vi "dds_reset.vi"(4 "constants in":T3, 7 "counter in":u8, 8 "FPGA parameters in":T2 {"y-point bandwidth" format="%.28g"; "x-point bandwidth" format="%.28g"; "AOD center frequ. (Hz)_y" format="%.14g"; "AOD half bandwidth_y" format="%.14g"; "AOD Bandwidth_y (Hz)" format="%_6f"; "AOD center frequ. (Hz)_x" format="%.14g"; "cos Phi" format="%.35g"; "sin Phi" format="%.35g"; "AOD_Scale_Factor (1/Zoom)" format="%.35g"; "AOD half bandwidth_x" format="%.14g"; "AOD Bandwidth_x (Hz)" format="%_6f"}, 9 "reset dds in":bool=TRUE, 10 "FPGA parameters after reset":T2 {"y-point bandwidth" format="%.28g"; "x-point bandwidth" format="%.28g"; "AOD center frequ. (Hz)_y" format="%.14g"; "AOD half bandwidth_y" format="%.14g"; "AOD Bandwidth_y (Hz)" format="%_6f"; "AOD center frequ. (Hz)_x" format="%.14g"; "cos Phi" format="%.35g"; "sin Phi" format="%.35g"; "AOD_Scale_Factor (1/Zoom)" format="%.35g"; "AOD half bandwidth_x" format="%.14g"; "AOD Bandwidth_x (Hz)" format="%_6f"}, 11 "synthesizer point in":T1) -> (0 "FPGA parameters out":T2 {"y-point bandwidth" format="%.28g"; "x-point bandwidth" format="%.28g"; "AOD center frequ. (Hz)_y" format="%.14g"; "AOD half bandwidth_y" format="%.14g"; "AOD Bandwidth_y (Hz)" format="%_6f"; "AOD center frequ. (Hz)_x" format="%.14g"; "cos Phi" format="%.35g"; "sin Phi" format="%.35g"; "AOD_Scale_Factor (1/Zoom)" format="%.35g"; "AOD half bandwidth_x" format="%.14g"; "AOD Bandwidth_x (Hz)" format="%_6f"}, 1 "reset dds out":bool, 3 "synthesizer point out":T1)   [LabVIEW 2010]
uses:
  FPGA_constants_cluster.ctl
  FPGA_parameters_cluster.ctl
  synthesizer_point_cluster.ctl
  <vilib>/eio/EIONode/EIONode.xnode
  <vilib>/rvi/eio/nirviEIOImplementation/nirviEIOImplementation.xnode
  <vilib>/rvi/eio/common/nirviEmuClasses.ctl
  <vilib>/rvi/eio/common/nirviEmuTemplateMethod_noerrors.vi
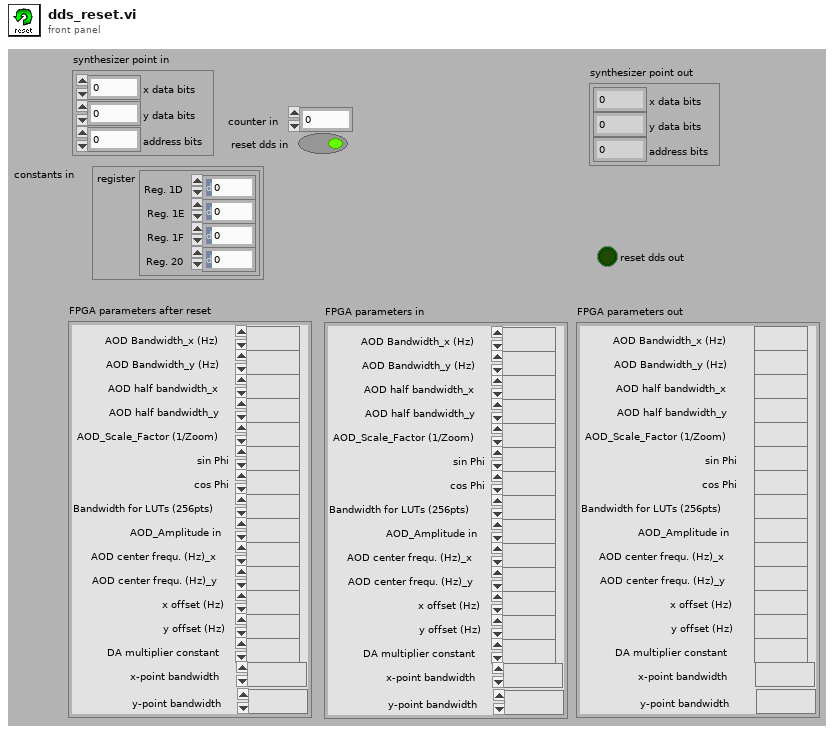
[diagram p1: front panel]
types:
  T1 = typedef "synthesizer_point_cluster.ctl" = cluster{"x data bits":u8, "y data bits":u8, "address bits":u8}
  T2 = typedef "FPGA_parameters_cluster.ctl" = cluster{"AOD Bandwidth_x (Hz)":fxp<+,36,32>, "AOD Bandwidth_y (Hz)":fxp<+,36,32>, "AOD half bandwidth_x":fxp<+,36,32>, "AOD half bandwidth_y":fxp<+,36,32>, "AOD_Scale_Factor (1/Zoom)":fxp<+,36,2>, "sin Phi":fxp<+/-,36,2>, "cos Phi":fxp<+/-,36,2>, "Bandwidth for LUTs (256pts)":fxp<+,36,0>, "AOD_Amplitude in":u16, "AOD center frequ. (Hz)_x":fxp<+,36,32>, "AOD center frequ. (Hz)_y":fxp<+,36,32>, "x offset (Hz)":fxp<+/-,36,32>, "y offset (Hz)":fxp<+/-,36,32>, "DA multiplier constant":fxp<+,64,4>, "x-point bandwidth":fxp<+,36,32>, "y-point bandwidth":fxp<+,36,32>}
  T3 = typedef "FPGA_constants_cluster.ctl" = cluster{"register":cluster{"Reg. 1D":u8, "Reg. 1E":u8, "Reg. 1F":u8, "Reg. 20":u8}}
  T4 = typedef "nirviEmuClasses.ctl" = enum16{"IO Read", "IO Write", "Method", "Property Read", "Property Write"}
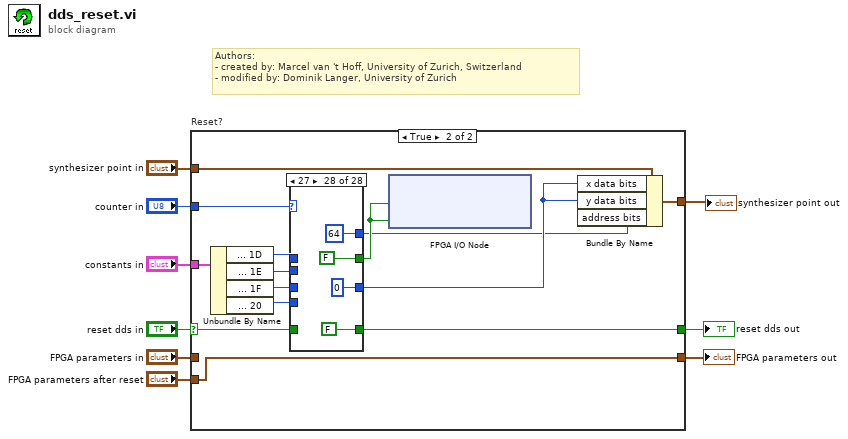
[diagram p0: block diagram]
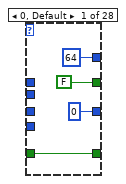
[diagram p3: hidden frame]
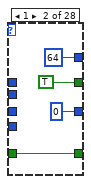
[diagram p4: hidden frame]
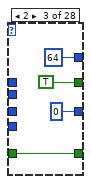
[diagram p5: hidden frame]
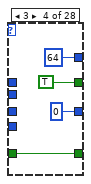
[diagram p6: hidden frame]
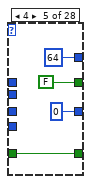
[diagram p7: hidden frame]
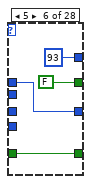
[diagram p8: hidden frame]
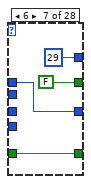
[diagram p9: hidden frame]
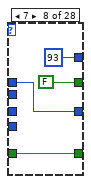
[diagram p10: hidden frame]
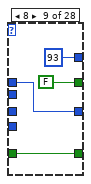
[diagram p11: hidden frame]
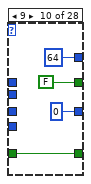
[diagram p12: hidden frame]
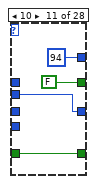
[diagram p13: hidden frame]
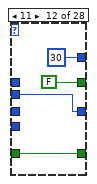
[diagram p14: hidden frame]
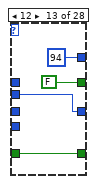
[diagram p15: hidden frame]
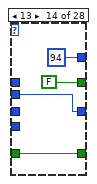
[diagram p16: hidden frame]
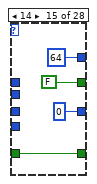
[diagram p17: hidden frame]
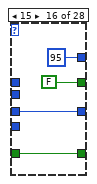
[diagram p18: hidden frame]
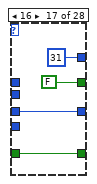
[diagram p19: hidden frame]
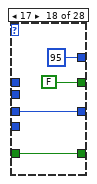
[diagram p20: hidden frame]
diagram:
  # "Authors: \n- created by: Marcel van 't Hoff, University of Zurich, Switzerland\n- modified by: Dominik Langer, University of Zurich"
  n1 = case "Reset?" shown="True" "reset dds in" {
    selector: "reset dds in" -> [w12 w19]
    tunnel: [w12 w18] -> w8
    tunnel: "constants in" -> [_ w22]
    tunnel: "counter in" -> [_ w20]
    tunnel: [w11 w17] -> w4
    tunnel: "FPGA parameters in" -> [w11 _]
    tunnel: "FPGA parameters after reset" -> [_ w17]
    tunnel: "synthesizer point in" -> [w10 w16]
    tunnel: [w10 w15] -> w1
    frame False {
    }
    frame True {
      n2 = Unbundle By Name(w22) -> ("register.Reg. 1D"=w23:u8, "register.Reg. 1E"=w24:u8, "register.Reg. 1F"=w25:u8, "register.Reg. 20"=w26:u8)
      n3 = case shown="27" w20 {
        tunnel: [u8 64 u8 64 u8 64 u8 64 u8 64 u8 93 u8 29 u8 93 u8 93 u8 64 u8 94 u8 30 u8 94 u8 94 u8 64 u8 95 u8 31 u8 95 u8 95 u8 64 u8 96 u8 32 u8 96 u8 96 u8 64 u8 64 u8 64 u8 64] -> w13
        tunnel: [u8 0 u8 0 u8 0 u8 0 u8 0 w72 w76 w80 w82 u8 0 w92 w96 w100 w102 u8 0 w112 w116 w120 w122 u8 0 w132 w136 w140 w142 u8 0 u8 0 u8 0 u8 0] -> w14
        tunnel: [FALSE TRUE TRUE TRUE FALSE FALSE FALSE FALSE FALSE FALSE FALSE FALSE FALSE FALSE FALSE FALSE FALSE FALSE FALSE FALSE FALSE FALSE FALSE FALSE FALSE FALSE FALSE FALSE] -> w21
        tunnel: w23 -> [_ _ _ _ _ w72 w76 w80 w82 _ _ _ _ _ _ _ _ _ _ _ _ _ _ _ _ _ _ _]
        tunnel: w24 -> [_ _ _ _ _ _ _ _ _ _ w92 w96 w100 w102 _ _ _ _ _ _ _ _ _ _ _ _ _ _]
        tunnel: w25 -> [_ _ _ _ _ _ _ _ _ _ _ _ _ _ _ w112 w116 w120 w122 _ _ _ _ _ _ _ _ _]
        tunnel: w26 -> [_ _ _ _ _ _ _ _ _ _ _ _ _ _ _ _ _ _ _ _ w132 w136 w140 w142 _ _ _ _]
        tunnel: w19 -> [w49 w53 w57 w61 w65 w69 w73 w77 w81 w85 w89 w93 w97 w101 w105 w109 w113 w117 w121 w125 w129 w133 w137 w141 w145 w149 w153 _]
        tunnel: [w49 w53 w57 w61 w65 w69 w73 w77 w81 w85 w89 w93 w97 w101 w105 w109 w113 w117 w121 w125 w129 w133 w137 w141 w145 w149 w153 FALSE] -> w18
        frame 0, Default {
        }
        frame 1 {
        }
        frame 2 {
        }
        frame 3 {
        }
        frame 4 {
        }
        frame 5 {
        }
        frame 6 {
        }
        frame 7 {
        }
        frame 8 {
        }
        frame 9 {
        }
        frame 10 {
        }
        frame 11 {
        }
        frame 12 {
        }
        frame 13 {
        }
        frame 14 {
        }
        frame 15 {
        }
        frame 16 {
        }
        frame 17 {
        }
        frame 18 {
        }
        frame 19 {
        }
        frame 20 {
        }
        frame 21 {
        }
        frame 22 {
        }
        frame 23 {
        }
        frame 24 {
        }
        frame 25 {
        }
        frame 26 {
        }
        frame 27 {
        }
      }
      n4 = xnode "FPGA I/O Node"("Connector3/DIO38"=w21, "Connector3/DIO39"=w21) -> ()  [unwired: 2 in, 2 out]
      n5 = Bundle By Name(cluster=w16, "x data bits"=w14, "y data bits"=w14, "address bits"=w13) -> (w15:T1)
    }
  }
  "reset dds out" <- w8
  "FPGA parameters out" <- w4
  "synthesizer point out" <- w1
